vi "NFScanPositionDefinition.vi"(3 "Width X (mm)":dbl=16.0, 11 "Max Frequency":dbl) -> ()   [LabVIEW 2017]
doc: "Use this template to build a user interface event handler design pattern. Use this pattern for dialog boxes and other user interfaces. You also can create and execute user-defined events that the VI can handle the same way as user interface events."
panel:
  out "i":i32
  out "Array":dbl[][](array[numeric])
  in  "OK Button":bool
  in  "Center Y (mm)":dbl
  in  "Center X (mm)":dbl
  in  "Pts in Y":dbl
  in  "Pts in X":dbl
  in  "dY (mm)":dbl
  in  "dX (mm)":dbl
  out "Span Y (mm)":dbl
  out "Span X (mm)":dbl
  in  "BtnGenerate":bool
  in  "Probe/AUT distance":dbl=12.0
  in  "Max FF angle (deg)":dbl=45.0
  in  "Height Y (mm)":dbl=16.0
  # "Scan Dimensions"
  # "AUT Dimensions"
  # "Delta"
  # "Scan center"
  # "Nbr of points"
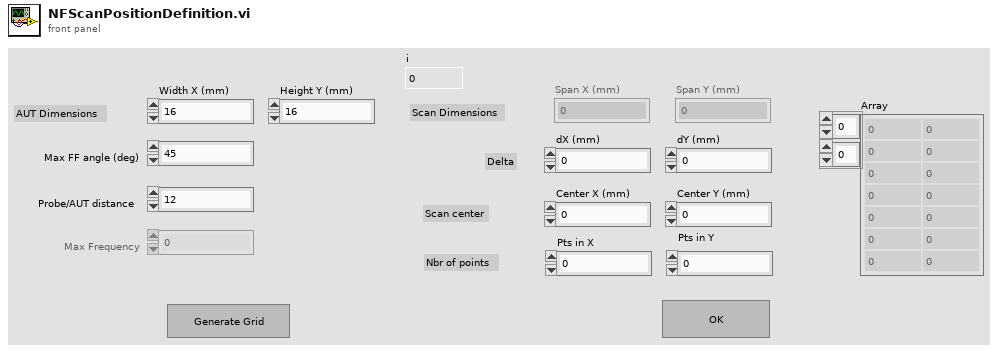
[diagram p1: front panel]
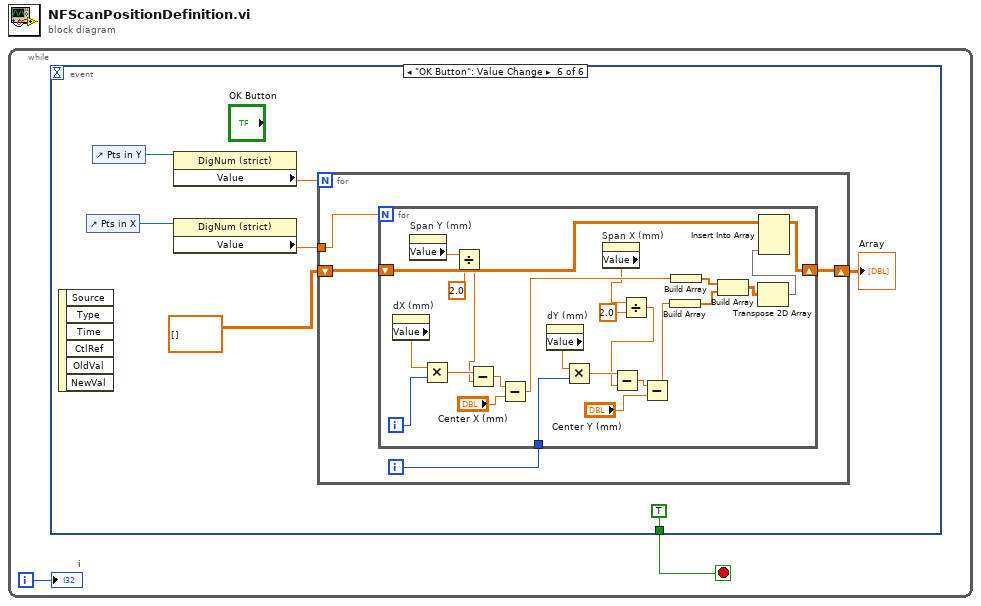
[diagram p0: block diagram]
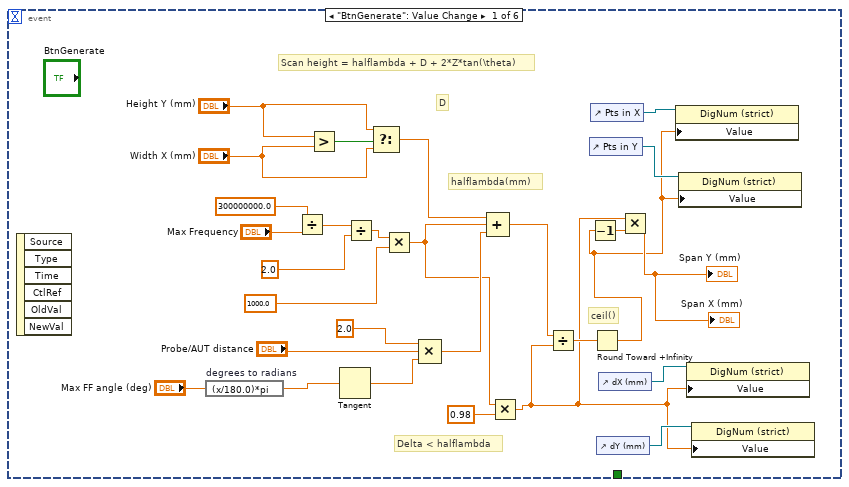
[diagram p2: hidden frame]
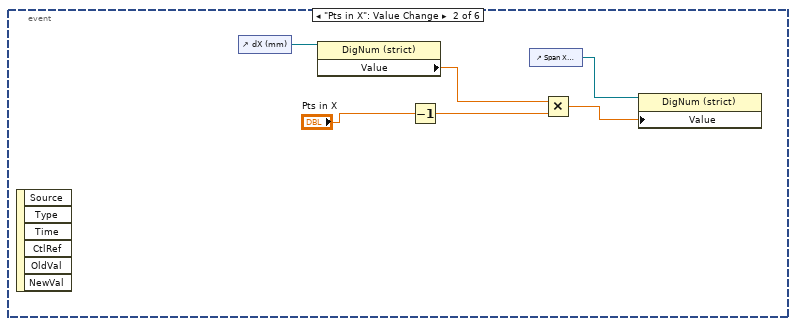
[diagram p3: hidden frame]
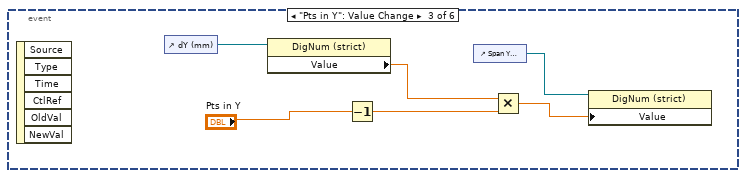
[diagram p4: hidden frame]
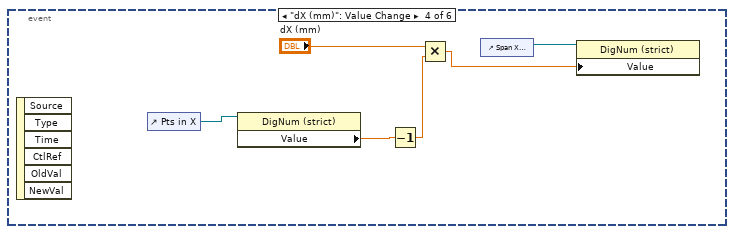
[diagram p5: hidden frame]
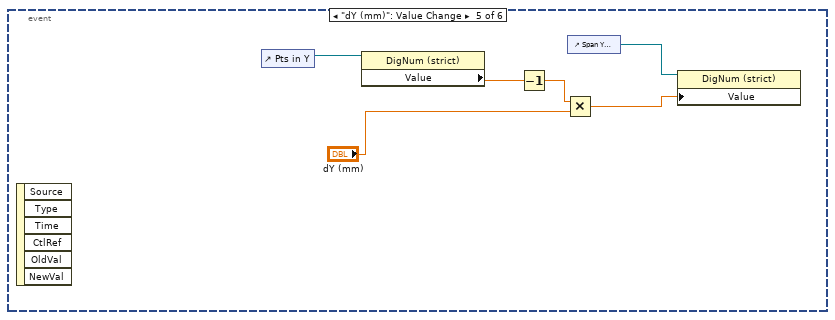
[diagram p6: hidden frame]
diagram:
  n1 = while {
    i -> [w1]
    stop <- w2 stop-if-true
    n2 = event shown="[5] \"OK Button\": Value Change" {
      selector: _ -> [_ _ _ _ _ _]
      dyn-events: _ -> [_ _ _ _ _ _]
      timeout: _ -> [_ _ _ _ _ _]
      tunnel: [_ _ _ _ _ TRUE ("stop")] -> w2
      event "BtnGenerate": Value Change {
        # "ceil()"
        # "Delta < halflambda"
        # "halflambda(mm)"
        # "D"
        # "Scan height = halflambda + D + 2*Z*tan(\\theta)"
        n3 = event-data() -> ()  [unwired: 1 in, 6 out]
        n4 = expression code="(x/180.0)*pi" "degrees to radians"("Max FF angle (deg)") -> (w6:dbl)
        n5 = Divide(x=300000000.0, y="Max Frequency") -> (x/y=w26:dbl)
        n6 = Greater?(x="Height Y (mm)", y="Width X (mm)") -> (0:w30:bool)
        n7 = Tangent(1:w6) -> (0:w22:dbl)
        n8 = Divide(x=w26, y=2.0) -> (x/y=w24:dbl)
        n9 = Select(t="Height Y (mm)", s=w30, f="Width X (mm)") -> (s? t:f=w29:dbl)
        n10 = Multiply(x=w24, y=1000.0) -> (x*y=w16:dbl)
        n11 = Compound Arithmetic op=MULTIPLY(2.0 ("value"), "Probe/AUT distance", w22) -> (w19:dbl)
        n12 = Compound Arithmetic op=ADD(w29, w16, w19) -> (w14:dbl)
        n13 = Multiply(x=w16, y=0.98) -> (x*y=w8:dbl)
        n14 = Divide(x=w14, y=w8) -> (x/y=w13:dbl)
        n15 = control-ref of="Pts in Y"() -> (w11:refnum<vi>)
        n16 = control-ref of="Pts in X"() -> (w12:refnum<vi>)
        n17 = Round Toward +Infinity(x=w13) -> (ceil(x): smallest int >= x=w3:dbl)
        n18 = Decrement(x=w3) -> (x-1=w4:dbl)
        n19 = control-ref of="dY (mm)"() -> (w9:refnum<vi>)
        n20 = control-ref of="dX (mm)"() -> (w10:refnum<vi>)
        n21 = Multiply(x=w8, y=w4) -> (x*y=→"Span Y (mm)" →"Span X (mm)":dbl)
        n22 = property class="DigNum (strict)"(reference=w12, "Value"=w3) -> ()  [unwired: 1 in, 2 out]
        n23 = property class="DigNum (strict)"(reference=w11, "Value"=w3) -> ()  [unwired: 1 in, 2 out]
        n24 = property class="DigNum (strict)"(reference=w10, "Value"=w8) -> ()  [unwired: 1 in, 2 out]
        n25 = property class="DigNum (strict)"(reference=w9, "Value"=w8) -> ()  [unwired: 1 in, 2 out]
      }
      event "Pts in X": Value Change {
        n26 = event-data() -> ()  [unwired: 1 in, 6 out]
        n27 = control-ref of="dX (mm)"() -> (w36:refnum<vi>)
        n28 = property class="DigNum (strict)"(reference=w36) -> ("Value"=w35:dbl)  [unwired: 1 in, 2 out]
        n29 = Decrement(x="Pts in X") -> (x-1=w32:dbl)
        n30 = control-ref of="Span X (mm)"() -> (w33:refnum<vi>)
        n31 = Multiply(x=w35, y=w32) -> (x*y=w34:dbl)
        n32 = property class="DigNum (strict)"(reference=w33, "Value"=w34) -> ()  [unwired: 1 in, 2 out]
      }
      event "Pts in Y": Value Change {
        n33 = event-data() -> ()  [unwired: 1 in, 6 out]
        n34 = control-ref of="dY (mm)"() -> (w39:refnum<vi>)
        n35 = property class="DigNum (strict)"(reference=w39) -> ("Value"=w41:dbl)  [unwired: 1 in, 2 out]
        n36 = Decrement(x="Pts in Y") -> (x-1=w37:dbl)
        n37 = control-ref of="Span Y (mm)"() -> (w40:refnum<vi>)
        n38 = Multiply(x=w41, y=w37) -> (x*y=w42:dbl)
        n39 = property class="DigNum (strict)"(reference=w40, "Value"=w42) -> ()  [unwired: 1 in, 2 out]
      }
      event "dX (mm)": Value Change {
        n40 = event-data() -> ()  [unwired: 1 in, 6 out]
        n41 = control-ref of="Pts in X"() -> (w47:refnum<vi>)
        n42 = property class="DigNum (strict)"(reference=w47) -> ("Value"=w44:dbl)  [unwired: 1 in, 2 out]
        n43 = Decrement(x=w44) -> (x-1=w43:dbl)
        n44 = Multiply(x="dX (mm)", y=w43) -> (x*y=w45:dbl)
        n45 = control-ref of="Span X (mm)"() -> (w46:refnum<vi>)
        n46 = property class="DigNum (strict)"(reference=w46, "Value"=w45) -> ()  [unwired: 1 in, 2 out]
      }
      event "dY (mm)": Value Change {
        n47 = event-data() -> ()  [unwired: 1 in, 6 out]
        n48 = control-ref of="Pts in Y"() -> (w54:refnum<vi>)
        n49 = property class="DigNum (strict)"(reference=w54) -> ("Value"=w51:dbl)  [unwired: 1 in, 2 out]
        n50 = Decrement(x=w51) -> (x-1=w50:dbl)
        n51 = Multiply(x=w50, y="dY (mm)") -> (x*y=w52:dbl)
        n52 = control-ref of="Span Y (mm)"() -> (w53:refnum<vi>)
        n53 = property class="DigNum (strict)"(reference=w53, "Value"=w52) -> ()  [unwired: 1 in, 2 out]
      }
      event "OK Button": Value Change {
        n54 = event-data() -> ()  [unwired: 1 in, 6 out]
        n55 = control-ref of="Pts in X"() -> (w58:refnum<vi>)
        n56 = control-ref of="Pts in Y"() -> (w57:refnum<vi>)
        n57 = property class="DigNum (strict)"(reference=w57) -> ("Value"=w61:dbl)  [unwired: 1 in, 2 out]
        n58 = property class="DigNum (strict)"(reference=w58) -> ("Value"=w59:dbl)  [unwired: 1 in, 2 out]
        n59 = for {
          N: w61 -> [_]
          tunnel: w59 -> [w65]
          shift-right: [w62] -> w55
          shift-left: dbl[][] [] -> [w63]
          i -> [w64]
          n60 = for {
            N: w65 -> [_]
            tunnel: w64 -> [w85]
            shift-right: [w78] -> w62
            shift-left: w63 -> [w79]
            i -> [w89]
            n61 = property on="dX (mm)" class="DigNum (strict)"() -> ("Value"=w88:dbl)  [unwired: 2 in, 2 out]
            n62 = property on="Span Y (mm)" class="DigNum (strict)"() -> ("Value"=w77:dbl)  [unwired: 2 in, 2 out]
            n63 = Multiply(x=w88, y=w89) -> (x*y=w69:dbl)
            n64 = Divide(x=w77, y=2.0) -> (x/y=w68:dbl)
            n65 = Subtract(x=w69, y=w68) -> (x-y=w70:dbl)
            n66 = Subtract(x=w70, y="Center X (mm)") -> (x-y=w82:dbl)
            n67 = property on="dY (mm)" class="DigNum (strict)"() -> ("Value"=w86:dbl)  [unwired: 2 in, 2 out]
            n68 = Multiply(x=w86, y=w85) -> (x*y=w67:dbl)
            n69 = property on="Span X (mm)" class="DigNum (strict)"() -> ("Value"=w74:dbl)  [unwired: 2 in, 2 out]
            n70 = Divide(x=w74, y=2.0) -> (x/y=w66:dbl)
            n71 = Subtract(x=w67, y=w66) -> (x-y=w75:dbl)
            n72 = Subtract(x=w75, y="Center Y (mm)") -> (x-y=w83:dbl)
            n73 = Build Array(w83) -> (w80:dbl[])
            n74 = Build Array(w82) -> (w81:dbl[])
            n75 = Build Array(w81, w80) -> (w72:dbl[][])
            n76 = Transpose 2D Array(2D array=w72) -> (transposed array=w71:dbl[][])
            n77 = Insert Into Array(array=w79, new element=w71) -> (w78:dbl[][])  [unwired: 2 in]
          }
        }
        "Array" <- w55
      }
    }
    "i" <- w1
  }
